vi "ReadBeamLineNode.vi"(8 "Error In":errorcluster, 11 "Experiment Node In":refnum<k20>) -> (0 "Error Out":errorcluster, 2 "Beam Line":T1={"Type"=enum."Ion Beam Analysis", "Ion"=enum."H", "Charge State"=0, "Total Source Ion Energy (kV)"=nan} {"Charge State" min=1}, 3 "Experiment Node Out":refnum<k20>)   [LabVIEW 2012]
uses:
  BeamLine.ctl
  BeamLineType.ctl
  BeamLineIon.ctl
  <vilib>/xml/NI_XML.lvlib
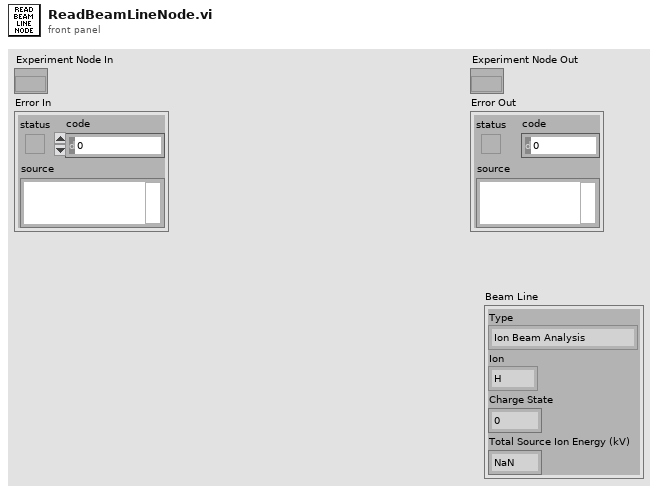
[diagram p1: front panel]
types:
  T1 = typedef "BeamLine.ctl" = cluster{"Type":T2, "Ion":T3, "Charge State":u8, "Total Source Ion Energy (kV)":dbl}
  T2 = typedef "BeamLineType.ctl" = enum16{"Ion Beam Analysis", "Auxiliary", "Radiation Damage"}
  T3 = typedef "BeamLineIon.ctl" = enum16{"H", "He", "C", "Fe", "Ni", "Pt", "Si", "Ag", "Au"}
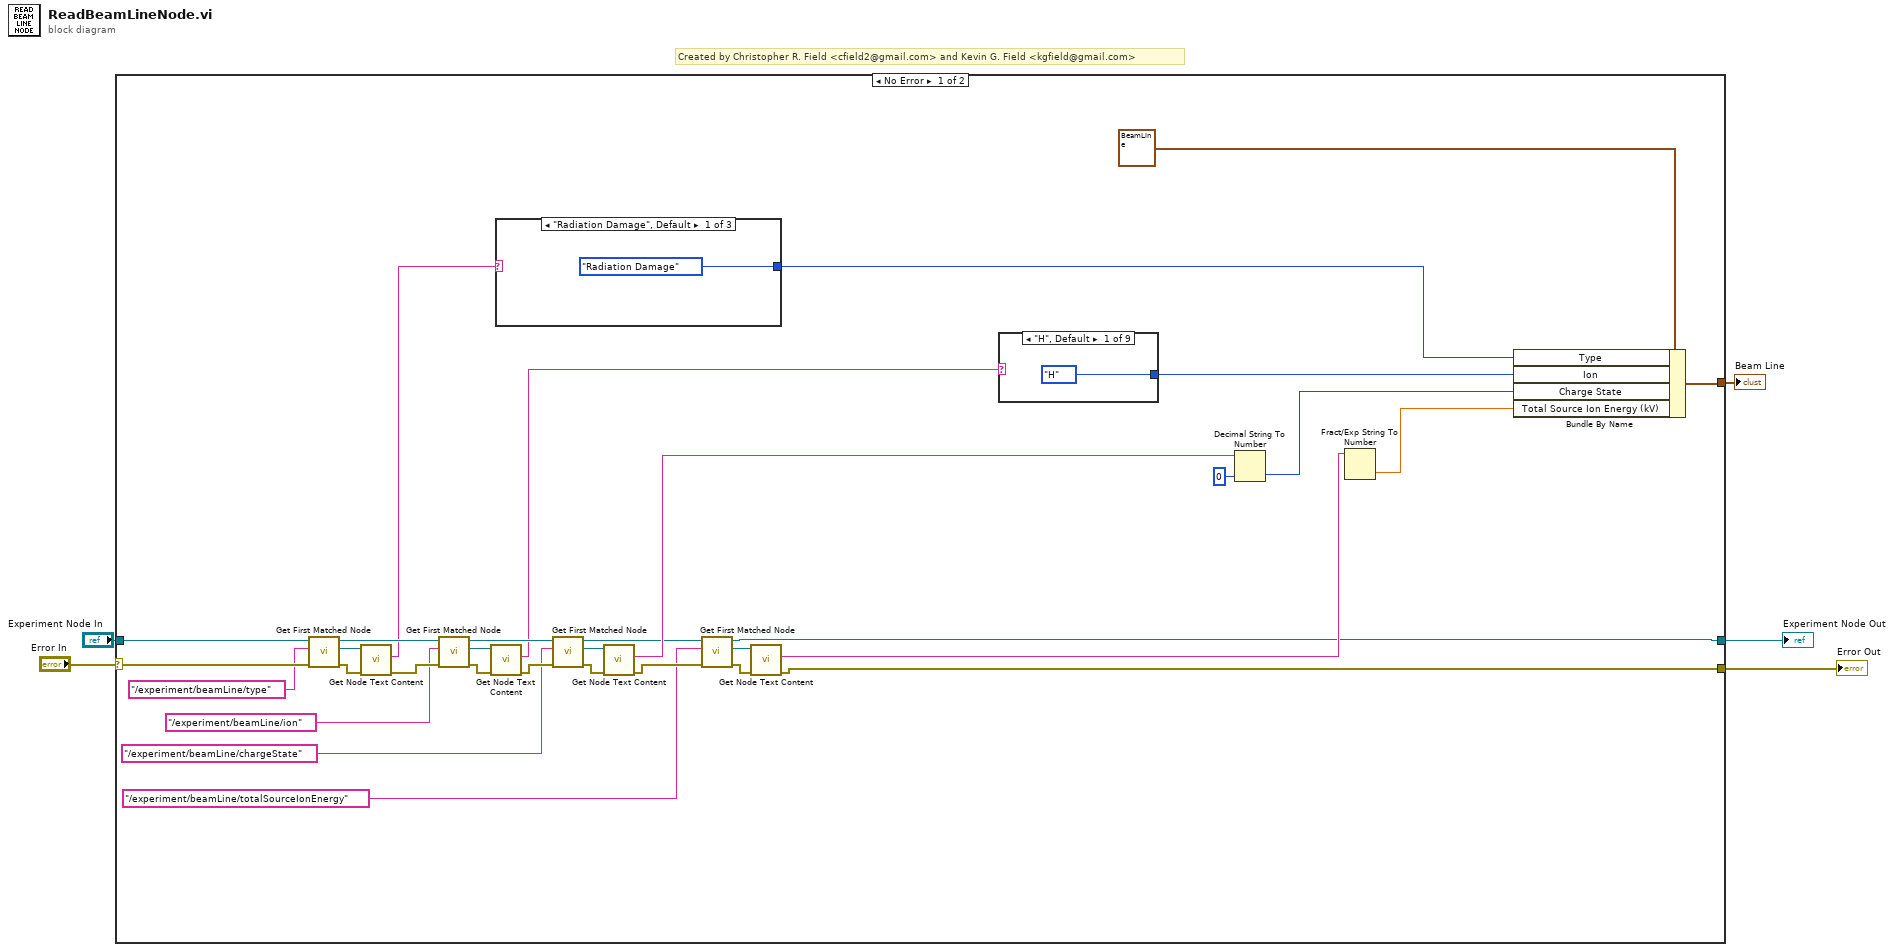
[diagram p0: block diagram]
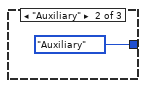
[diagram p2: hidden frame]
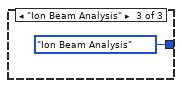
[diagram p3: hidden frame]
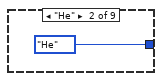
[diagram p4: hidden frame]
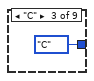
[diagram p5: hidden frame]
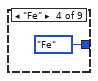
[diagram p6: hidden frame]
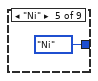
[diagram p7: hidden frame]
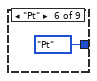
[diagram p8: hidden frame]
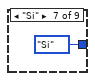
[diagram p9: hidden frame]
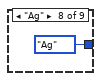
[diagram p10: hidden frame]
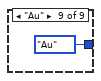
[diagram p11: hidden frame]
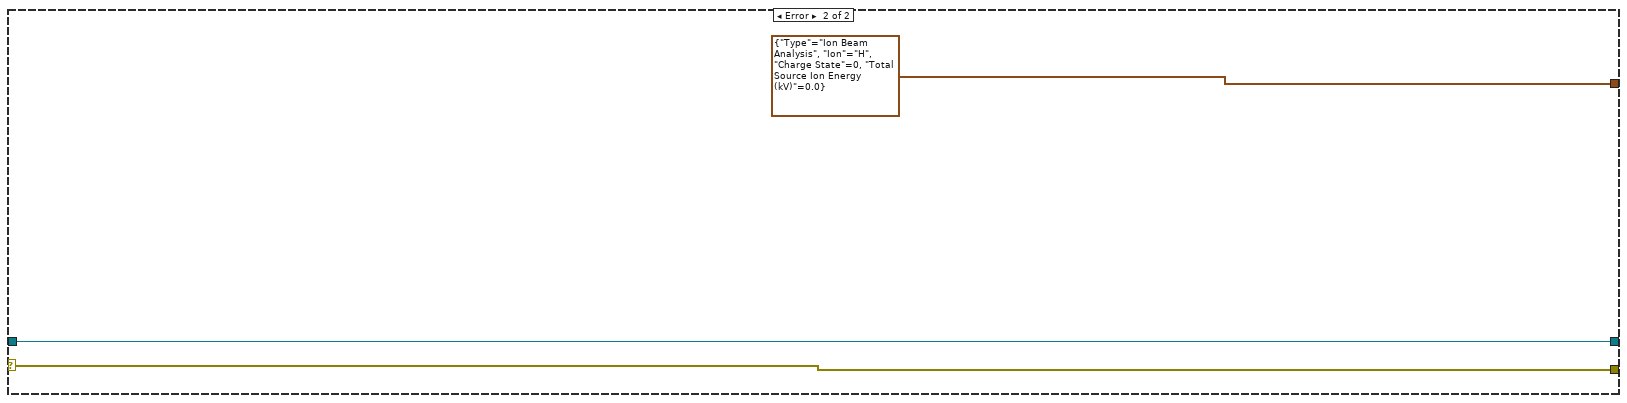
[diagram p12: hidden frame]
diagram:
  # "Created by Christopher R. Field <cfield2@gmail.com> and Kevin G. Field <kgfield@gmail.com>"
  n1 = case shown="No Error" "Error In" {
    selector: "Error In" -> [w37 w52]
    tunnel: "Experiment Node In" -> [w38 w53]
    tunnel: [w7 w53] -> w3
    tunnel: [w6 w52] -> w2
    tunnel: [w15 T1 {"Type"=enum."Ion Beam Analysis", "Ion"=enum."H", "Charge State"=0, "Total Source Ion Energy (kV)"=0.0} ("Beam Line")] -> w1
    frame No Error {
      n2 = call <vilib>:"Get First Matched Node.vi"("error in (no error)"=w37, "XPath expression"="/experiment/beamLine/type", "node in"=w38) -> ("error out"=w34:errorcluster, "node result"=w35:refnum<k20>, "node out"=w33:refnum<k20>)  [unwired: 6 in]
      n3 = call <vilib>:"Get Node Text Content.vi"("error in (no error)"=w34, "node in"=w35) -> ("error out"=w32:errorcluster, "node text"=w17:string)  [unwired: 7 in, 1 out]
      n4 = call <vilib>:"Get First Matched Node.vi"("error in (no error)"=w32, "XPath expression"="/experiment/beamLine/ion", "node in"=w33) -> ("error out"=w29:errorcluster, "node result"=w30:refnum<k20>, "node out"=w28:refnum<k20>)  [unwired: 6 in]
      n5 = call <vilib>:"Get Node Text Content.vi"("error in (no error)"=w29, "node in"=w30) -> ("error out"=w27:errorcluster, "node text"=w19:string)  [unwired: 7 in, 1 out]
      n6 = case shown="\"Radiation Damage\", Default" w17 {
        tunnel: [BeamLineType."Radiation Damage" ("Type") BeamLineType."Auxiliary" ("Type") BeamLineType."Ion Beam Analysis" ("Type")] -> w16
        frame "Radiation Damage", Default {
        }
        frame "Auxiliary" {
        }
        frame "Ion Beam Analysis" {
        }
      }
      n7 = call <vilib>:"Get First Matched Node.vi"("error in (no error)"=w27, "XPath expression"="/experiment/beamLine/chargeState", "node in"=w28) -> ("error out"=w24:errorcluster, "node result"=w25:refnum<k20>, "node out"=w14:refnum<k20>)  [unwired: 6 in]
      n8 = call <vilib>:"Get Node Text Content.vi"("error in (no error)"=w24, "node in"=w25) -> ("error out"=w13:errorcluster, "node text"=w22:string)  [unwired: 7 in, 1 out]
      n9 = call <vilib>:"Get First Matched Node.vi"("error in (no error)"=w13, "XPath expression"="/experiment/beamLine/totalSourceIonEnergy", "node in"=w14) -> ("error out"=w11:errorcluster, "node result"=w12:refnum<k20>, "node out"=w7:refnum<k20>)  [unwired: 6 in]
      n10 = call <vilib>:"Get Node Text Content.vi"("error in (no error)"=w11, "node in"=w12) -> ("error out"=w6:errorcluster, "node text"=w8:string)  [unwired: 7 in, 1 out]
      n11 = case shown="\"H\", Default" w19 {
        tunnel: [BeamLineIon."H" ("Ion") BeamLineIon."He" ("Ion") BeamLineIon."C" ("Ion") BeamLineIon."Fe" ("Ion") BeamLineIon."Ni" ("Ion") BeamLineIon."Pt" ("Ion") BeamLineIon."Si" ("Ion") BeamLineIon."Ag" ("Ion") BeamLineIon."Au" ("Ion")] -> w18
        frame "H", Default {
        }
        frame "He" {
        }
        frame "C" {
        }
        frame "Fe" {
        }
        frame "Ni" {
        }
        frame "Pt" {
        }
        frame "Si" {
        }
        frame "Ag" {
        }
        frame "Au" {
        }
      }
      n12 = Decimal String To Number(string=w22, default (0L)=u8 0 ("default (0 I32)")) -> (number=w20:u8)  [unwired: 1 in, 1 out]
      n13 = Fract/Exp String To Number(string=w8) -> (number=w9:dbl)  [unwired: 3 in, 1 out]
      n14 = Bundle By Name(cluster=T1 {"Type"=enum."Ion Beam Analysis", "Ion"=enum."H", "Charge State"=0, "Total Source Ion Energy (kV)"=0.0} ("Beam Line"), "Type"=w16, "Ion"=w18, "Charge State"=w20, "Total Source Ion Energy (kV)"=w9) -> (w15:T1)
    }
    frame Error {
    }
  }
  "Experiment Node Out" <- w3
  "Error Out" <- w2
  "Beam Line" <- w1
